vi "Example Loopback.vi"() -> ()   [LabVIEW 2013]
uses:
  C:/tf/play/labview/Tinkerforge.dll
  Tinkerforge.dll
panel:
  out "length":u8
  out "data":u8[](array[numeric])
  out "identifier":i64
  out "frameType":u8
  in  "stop":bool
  in  "uid":string="5556"
  in  "port":i32=4223
  in  "host":string="localhost"
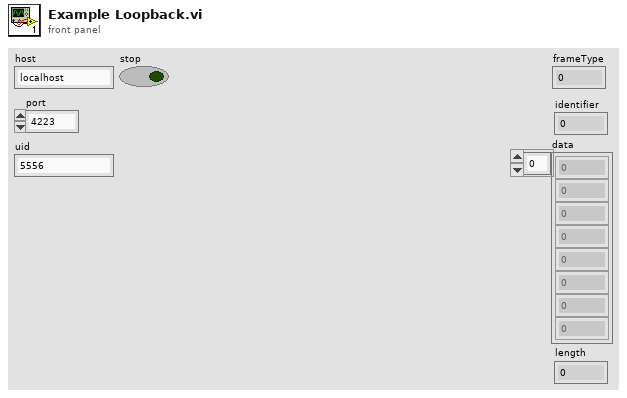
[diagram p1: front panel]
types:
  T1 = cluster{"data":u8[], "length":u8, "frameType":u8, "identifier":i64}
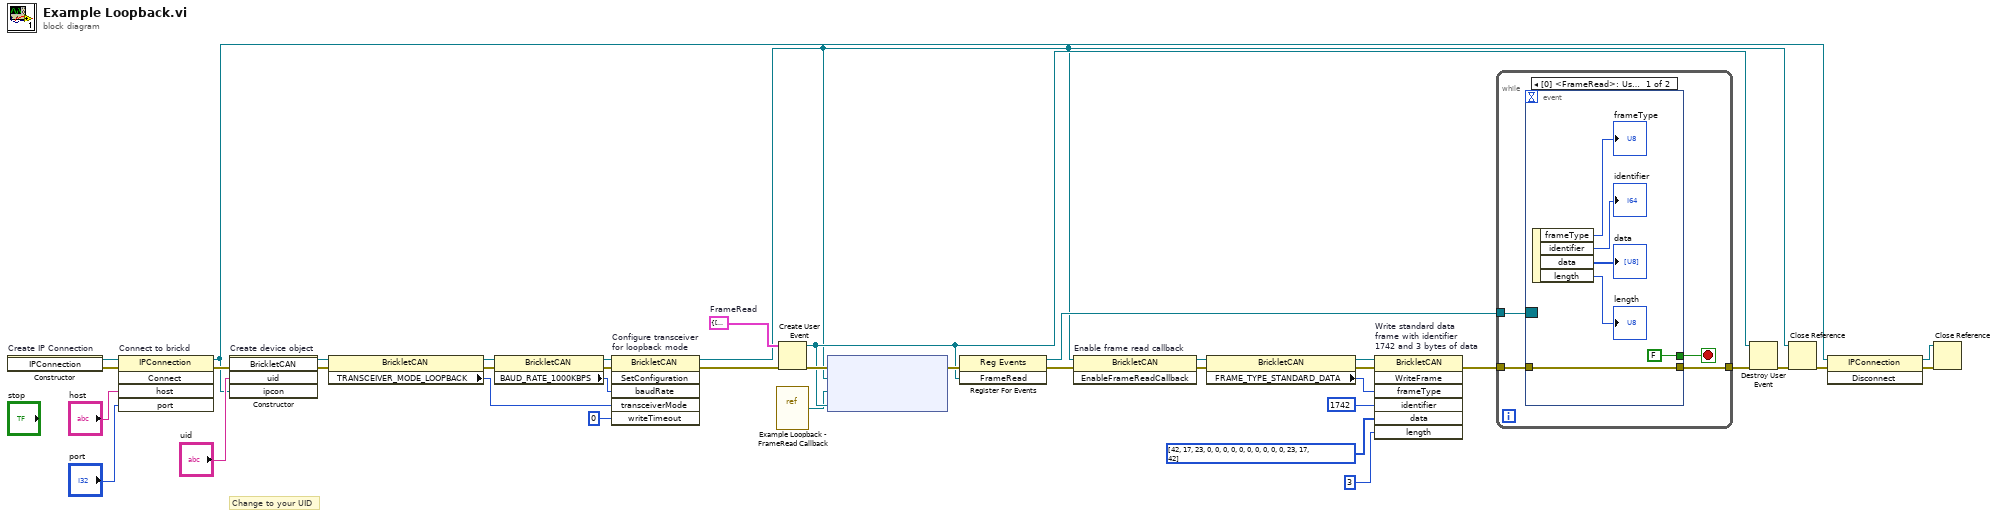
[diagram p0: block diagram]
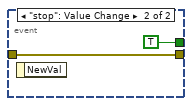
[diagram p2: hidden frame]
diagram:
  w23 = T1 {"data"=[], "length"=0, "frameType"=0, "identifier"=0}  # FrameRead
  # "Change to your UID"
  n1 = constructor on="Create IP Connection" class="IPConnection"() -> (reference out=w39:refnum<k24>, error out=w24:errorcluster)  [unwired: 3 in, 1 out]
  n2 = invoke on="Connect to brickd" class="IPConnection" method="Connect"(reference=w39, error in=w24, "host"="host", "port"="port") -> (reference out=w32:refnum<k24>, error out=w35:errorcluster)  [unwired: 1 in, 3 out]
  n3 = constructor on="Create device object" class="BrickletCAN"(error in=w35, "uid"="uid", "ipcon"=w32) -> (reference out=w5:refnum<k24>, error out=w6:errorcluster)  [unwired: 2 in, 3 out]
  n4 = property class="BrickletCAN"(reference=w5, error in=w6) -> (reference out=w8:refnum<k24>, error out=w10:errorcluster, "TRANSCEIVER_MODE_LOOPBACK"=w1:u8)
  n5 = property class="BrickletCAN"(reference=w8, error in=w10) -> (reference out=w7:refnum<k24>, error out=w9:errorcluster, "BAUD_RATE_1000KBPS"=w2:u8)
  n6 = invoke on="Configure transceiver\nfor loopback mode" class="BrickletCAN" method="SetConfiguration"(reference=w7, error in=w9, "baudRate"=w2, "transceiverMode"=w1, "writeTimeout"=0) -> (reference out=w4:refnum<k24>, error out=w3:errorcluster)  [unwired: 1 in, 4 out]
  n7 = vi-ref "Example Loopback - FrameRead Callback.vi"() -> ("vi reference"=w12:refnum<vi>)
  n8 = Create User Event(user event datatype=w23, error in=w3) -> (user event=w26:refnum<user-event>, error out=w30:errorcluster)
  n9 = node ("Register Event Callback")(w30, w4, w12, w26) -> (w29:errorcluster)  [unwired: 1 in, 1 out]
  n10 = register-events(error in=w29, w26) -> (reference out=w28:refnum<event-registration>, error out=w22:errorcluster)  [unwired: 1 in]
  n11 = invoke on="Enable frame read callback" class="BrickletCAN" method="EnableFrameReadCallback"(reference=w4, error in=w22) -> (reference out=w20:refnum<k24>, error out=w18:errorcluster)  [unwired: 1 in, 1 out]
  n12 = property class="BrickletCAN"(reference=w20, error in=w18) -> (reference out=w19:refnum<k24>, error out=w17:errorcluster, "FRAME_TYPE_STANDARD_DATA"=w16:u8)
  n13 = invoke on="Write standard data\nframe with identifier\n1742 and 3 bytes of data" class="BrickletCAN" method="WriteFrame"(reference=w19, error in=w17, "frameType"=w16, "identifier"=i64 1742, "data"=u8[] [42, 17, 23, 0, 0, 0, 0, 0, 0, 0, 0, 0, 0, 23, 17, 42], "length"=u8 3) -> (error out=w21:errorcluster)  [unwired: 1 in, 6 out]
  n14 = while {
    tunnel: w28 -> [w43]
    tunnel: [w42] -> w27
    tunnel: w21 -> [w41]
    stop <- w40 stop-if-true
    n15 = event shown="[0] <FrameRead>: User Event" {
      selector: w43 -> [_ _]
      dyn-events: _ -> [_ _]
      timeout: _ -> [_ _]
      tunnel: [w49 w50] -> w42
      tunnel: w41 -> [w49 w50]
      tunnel: [FALSE TRUE] -> w40
      event User Event {
        n16 = event-data() -> ("frameType"=→"frameType":u8, "identifier"=→"identifier":i64, "data"=→"data":u8[], "length"=→"length":u8)  [unwired: 1 in]
      }
      event "stop": Value Change {
        n17 = event-data() -> ()  [unwired: 1 in, 1 out]
      }
    }
  }
  n18 = Destroy User Event(user event=w26, error in=w27) -> (error out=w25:errorcluster)
  n19 = Close Reference(reference=w4, error in (no error)=w25) -> (error out=w34:errorcluster)
  n20 = invoke class="IPConnection" method="Disconnect"(reference=w32, error in=w34) -> (reference out=w31:refnum<k24>, error out=w33:errorcluster)  [unwired: 1 in, 1 out]
  n21 = Close Reference(reference=w31, error in (no error)=w33) -> ()  [unwired: 1 out]
